vi "TCam_Config.vi"(8 "error in (no error)":errorcluster, 10 "crop?":bool, 11 "DataCluster in":T1={"Core"={"Current VI Reference"=refnum, "Close Panel on Exit?"=FALSE, "Exit"=FALSE, "Initialized?"=FALSE}, "Connections"={"cDAQ"={"Task"="", "Connected"=FALSE, "Active"=FALSE, "ID"=""}, "Camera"={"Session"="", "Connected"=FALSE, "Active"=FALSE, "Placeholder"=refnum}, "PSU"={"Port"="", "Connected"=FALSE, "Active"=FALSE}, "Arduino"={"Port"="", "Connected"=FALSE, "Active"=FALSE}}, "Data Acquisition"={"Setup"={"Label"="", "Operator"="", "Notes"="", "TempGrad"=1.0, "TargetTemp"=1.0, "Sample Volume"=1.0}, "Camera"={"Image"=refnum, "Save Image"=refnum, "Image Frequency"=20, "Rectangle"={"Left"=0, "Top"=0, "Right"=0, "Bottom"=0, "Rotation"=0.0}, "Calibration"={"Top Left"={"X"=0.0, "Y"=0.0}, "Top Right"={"X"=0.0, "Y"=0.0}, "Bottom Left"={"X"=0.0, "Y"=0.0}, "Bottom Right"={"X"=0.0, "Y"=0.0}, "Fixpoint"={"X"=0.0, "Y"=0.0}, "Scan Area"=0.0, "Fixpoint Area"=0.0, "Well Pixels"=[], "Valid"=FALSE}, "FocusPos"=0, "Display Mapping"=10, "Camera Mode"=10}, "Thermistor"={"Sample Size"=1, "Calibration"={"B0.100"=[], "R25"=[], "c"=[], "State"=[], "V_S"=5.0, "R_S"=100.0}, "Timing Mode"=14713}, "Partition"={"Data"=[], "Cell Label"="", "Cell Color"=0, "Height"=10, "Width"=16, "Grid"=[]}, "Queue"={"Size"=1, "Queue"=refnum}, "Sample Rate"=1, "Active"=FALSE, "Ready"=FALSE, "Graph Mode"=0, "Gradient Buffer"=2}, "Control"={"Sample Rate"=1, "PID gains"={"proportional gain (Kc)"=1.0, "integral time (Ti, min)"=0.01, "derivative time (Td, min)"=0.0}}, "Manual Temp Control"={"TargetTemp"=1.0, "Mode"=0, "Active"=FALSE}} {"Manual Temp Control"."Mode" items=["Cool", "Heat"]; "Manual Temp Control"."TargetTemp" min=-40.0 max=40.0 step=0.5 format="%#_g °C"; "Control"."PID gains"."derivative time (Td, min)" format="%.3f"; "Control"."PID gains"."integral time (Ti, min)" format="%.3f"; "Control"."PID gains"."proportional gain (Kc)" format="%.3f"; "Control"."Sample Rate" min=1 max=20 step=1 format="%.0f Samples/sec"; "Data Acquisition"."Gradient Buffer" min=2 max=30 step=1; "Data Acquisition"."Graph Mode" items=["Thermistor Temperature", "Camera Temperature"]; "Data Acquisition"."Thermistor"."Timing Mode" items=["Automatic"=16097, "High Resolution"=10195, "High Speed"=14712, "Best 50 Hz Rejection"=14713, "Best 60 Hz Rejection"=14714, "Custom"=10137]; "Data Acquisition"."Thermistor"."Calibration"."R_S" min=0.1 max=1000.0 format="%#_g kOhm"; "Data Acquisition"."Thermistor"."Calibration"."V_S" min=5.0 max=48.0 format="%#_g V"; "Data Acquisition"."Thermistor"."Calibration"."R25" min=0.1 max=1000.0 format="%#_g kOhm"; "Data Acquisition"."Thermistor"."Calibration"."B0.100" min=100.0 max=10000.0 format="%#_g K"; "Data Acquisition"."Thermistor"."Sample Size" min=1 max=200; "Data Acquisition"."Sample Rate" min=20 max=240 format="%.0f samples/min"; "Data Acquisition"."Queue"."Size" min=1 max=200; "Data Acquisition"."Camera"."Camera Mode" items=["Temperature Linear", "Signal Linear"]; "Data Acquisition"."Camera"."Display Mapping" items=["Default"=10, "Most Significant Bits"=11, "Full Dynamic"=12, "Downshift"=13, "Given Range"=14, "90% Dynamic"=15, "Given Percent Range"=16]; "Data Acquisition"."Camera"."Calibration"."Fixpoint"."Y" format="%.2f"; "Data Acquisition"."Camera"."Calibration"."Fixpoint"."X" format="%.2f"; "Data Acquisition"."Camera"."Calibration"."Top Left"."Y" format="%.2f"; "Data Acquisition"."Camera"."Calibration"."Top Left"."X" format="%.2f"; "Data Acquisition"."Camera"."Calibration"."Top Right"."Y" format="%.2f"; "Data Acquisition"."Camera"."Calibration"."Top Right"."X" format="%.2f"; "Data Acquisition"."Camera"."Calibration"."Bottom Left"."Y" format="%.2f"; "Data Acquisition"."Camera"."Calibration"."Bottom Left"."X" format="%.2f"; "Data Acquisition"."Camera"."Calibration"."Bottom Right"."Y" format="%.2f"; "Data Acquisition"."Camera"."Calibration"."Bottom Right"."X" format="%.2f"; "Data Acquisition"."Camera"."Rectangle"."Rotation" min=-90.0 max=90.0 step=1.0 format="%.2f"; "Data Acquisition"."Camera"."Rectangle"."Left" scale=0.0..1024.0; "Data Acquisition"."Camera"."Rectangle"."Right" scale=0.0..1024.0; "Data Acquisition"."Camera"."Image Frequency" min=1 max=60 step=1; "Data Acquisition"."Setup"."Sample Volume" min=0.0 max=500.0 format="%#_g µL"; "Data Acquisition"."Setup"."TargetTemp" min=-40.0 max=40.0 step=0.5 format="%#_g °C"; "Data Acquisition"."Setup"."TempGrad" min=-100.0 max=100.0 step=0.1 format="%#_g °C/min"}) -> (0 "error out":errorcluster, 3 "DataCluster out":T1={"Core"={"Current VI Reference"=refnum, "Close Panel on Exit?"=FALSE, "Exit"=FALSE, "Initialized?"=FALSE}, "Connections"={"cDAQ"={"Task"="", "Connected"=FALSE, "Active"=FALSE, "ID"=""}, "Camera"={"Session"="", "Connected"=FALSE, "Active"=FALSE, "Placeholder"=refnum}, "PSU"={"Port"="", "Connected"=FALSE, "Active"=FALSE}, "Arduino"={"Port"="", "Connected"=FALSE, "Active"=FALSE}}, "Data Acquisition"={"Setup"={"Label"="", "Operator"="", "Notes"="", "TempGrad"=1.0, "TargetTemp"=1.0, "Sample Volume"=1.0}, "Camera"={"Image"=refnum, "Save Image"=refnum, "Image Frequency"=20, "Rectangle"={"Left"=0, "Top"=0, "Right"=0, "Bottom"=0, "Rotation"=0.0}, "Calibration"={"Top Left"={"X"=0.0, "Y"=0.0}, "Top Right"={"X"=0.0, "Y"=0.0}, "Bottom Left"={"X"=0.0, "Y"=0.0}, "Bottom Right"={"X"=0.0, "Y"=0.0}, "Fixpoint"={"X"=0.0, "Y"=0.0}, "Scan Area"=0.0, "Fixpoint Area"=0.0, "Well Pixels"=[], "Valid"=FALSE}, "FocusPos"=0, "Display Mapping"=10, "Camera Mode"=10}, "Thermistor"={"Sample Size"=1, "Calibration"={"B0.100"=[], "R25"=[], "c"=[], "State"=[], "V_S"=5.0, "R_S"=100.0}, "Timing Mode"=14713}, "Partition"={"Data"=[], "Cell Label"="", "Cell Color"=0, "Height"=10, "Width"=16, "Grid"=[]}, "Queue"={"Size"=1, "Queue"=refnum}, "Sample Rate"=1, "Active"=FALSE, "Ready"=FALSE, "Graph Mode"=0, "Gradient Buffer"=2}, "Control"={"Sample Rate"=1, "PID gains"={"proportional gain (Kc)"=1.0, "integral time (Ti, min)"=0.01, "derivative time (Td, min)"=0.0}}, "Manual Temp Control"={"TargetTemp"=1.0, "Mode"=0, "Active"=FALSE}} {"Manual Temp Control"."Mode" items=["Cool", "Heat"]; "Manual Temp Control"."TargetTemp" min=-40.0 max=40.0 step=0.5 format="%#_g °C"; "Control"."PID gains"."derivative time (Td, min)" format="%.3f"; "Control"."PID gains"."integral time (Ti, min)" format="%.3f"; "Control"."PID gains"."proportional gain (Kc)" format="%.3f"; "Control"."Sample Rate" min=1 max=20 step=1 format="%.0f Samples/sec"; "Data Acquisition"."Gradient Buffer" min=2 max=30 step=1; "Data Acquisition"."Graph Mode" items=["Thermistor Temperature", "Camera Temperature"]; "Data Acquisition"."Thermistor"."Timing Mode" items=["Automatic"=16097, "High Resolution"=10195, "High Speed"=14712, "Best 50 Hz Rejection"=14713, "Best 60 Hz Rejection"=14714, "Custom"=10137]; "Data Acquisition"."Thermistor"."Calibration"."R_S" min=0.1 max=1000.0 format="%#_g kOhm"; "Data Acquisition"."Thermistor"."Calibration"."V_S" min=5.0 max=48.0 format="%#_g V"; "Data Acquisition"."Thermistor"."Calibration"."R25" min=0.1 max=1000.0 format="%#_g kOhm"; "Data Acquisition"."Thermistor"."Calibration"."B0.100" min=100.0 max=10000.0 format="%#_g K"; "Data Acquisition"."Thermistor"."Sample Size" min=1 max=200; "Data Acquisition"."Sample Rate" min=20 max=240 format="%.0f samples/min"; "Data Acquisition"."Queue"."Size" min=1 max=200; "Data Acquisition"."Camera"."Camera Mode" items=["Temperature Linear", "Signal Linear"]; "Data Acquisition"."Camera"."Display Mapping" items=["Default"=10, "Most Significant Bits"=11, "Full Dynamic"=12, "Downshift"=13, "Given Range"=14, "90% Dynamic"=15, "Given Percent Range"=16]; "Data Acquisition"."Camera"."Calibration"."Fixpoint"."Y" format="%.2f"; "Data Acquisition"."Camera"."Calibration"."Fixpoint"."X" format="%.2f"; "Data Acquisition"."Camera"."Calibration"."Top Left"."Y" format="%.2f"; "Data Acquisition"."Camera"."Calibration"."Top Left"."X" format="%.2f"; "Data Acquisition"."Camera"."Calibration"."Top Right"."Y" format="%.2f"; "Data Acquisition"."Camera"."Calibration"."Top Right"."X" format="%.2f"; "Data Acquisition"."Camera"."Calibration"."Bottom Left"."Y" format="%.2f"; "Data Acquisition"."Camera"."Calibration"."Bottom Left"."X" format="%.2f"; "Data Acquisition"."Camera"."Calibration"."Bottom Right"."Y" format="%.2f"; "Data Acquisition"."Camera"."Calibration"."Bottom Right"."X" format="%.2f"; "Data Acquisition"."Camera"."Rectangle"."Rotation" min=-90.0 max=90.0 step=1.0 format="%.2f"; "Data Acquisition"."Camera"."Rectangle"."Left" scale=0.0..1024.0; "Data Acquisition"."Camera"."Rectangle"."Right" scale=0.0..1024.0; "Data Acquisition"."Camera"."Image Frequency" min=1 max=60 step=1; "Data Acquisition"."Setup"."Sample Volume" min=0.0 max=500.0 format="%#_g µL"; "Data Acquisition"."Setup"."TargetTemp" min=-40.0 max=40.0 step=0.5 format="%#_g °C"; "Data Acquisition"."Setup"."TempGrad" min=-100.0 max=100.0 step=0.1 format="%#_g °C/min"})   [LabVIEW 2024]
uses:
  DataCluster.ctl
  <vilib>/userDefined/High Color/IMAQdx.ctl
  <vilib>/vision/Image Controls.llb/IMAQ Image.ctl
  <vilib>/vision/driver/IMAQdx.llb/IMAQdx Acquisition Mode.ctl
  05920238-52a0-44ea-981a-fd3a139130d6.vi
  <resource>/objmgr/imaqdx.rc
  <vilib>/vision/driver/NI_Vision_Acquisition_Software.lvlib
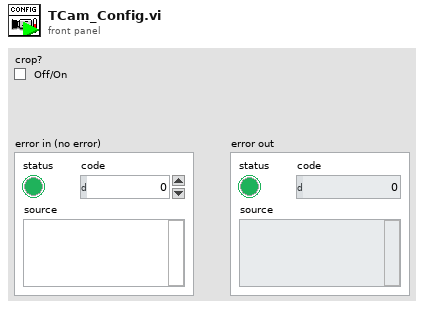
[diagram p1: front panel]
types:
  T1 = typedef "DataCluster.ctl" = cluster{"Core":cluster{"Current VI Reference":refnum<vi>, "Close Panel on Exit?":bool, "Exit":bool, "Initialized?":bool}, "Connections":cluster{"cDAQ":cluster{"Task":refnum<k21>, "Connected":bool, "Active":bool, "ID":string}, "Camera":cluster{"Session":T2, "Connected":bool, "Active":bool, "Placeholder":T3}, "PSU":cluster{"Port":refnum<visa-resource-name>, "Connected":bool, "Active":bool}, "Arduino":cluster{"Port":refnum<visa-resource-name>, "Connected":bool, "Active":bool}}, "Data Acquisition":cluster{"Setup":cluster{"Label":string, "Operator":string, "Notes":string, "TempGrad":dbl, "TargetTemp":dbl, "Sample Volume":dbl}, "Camera":cluster{"Image":T3, "Save Image":T3, "Image Frequency":i32, "Rectangle":T4, "Calibration":cluster{"Top Left":T5, "Top Right":T5, "Bottom Left":T5, "Bottom Right":T5, "Fixpoint":T5, "Scan Area":dbl, "Fixpoint Area":dbl, "Well Pixels":cluster{"X":i32, "Y":i32}[][], "Valid":bool}, "FocusPos":u32, "Display Mapping":u32, "Camera Mode":u32}, "Thermistor":cluster{"Sample Size":i32, "Calibration":cluster{"B0.100":dbl[], "R25":dbl[], "c":dbl[][], "State":bool[], "V_S":dbl, "R_S":dbl}, "Timing Mode":i32}, "Partition":cluster{"Data":string[][], "Cell Label":string, "Cell Color":u32, "Height":i32, "Width":i32, "Grid":string[][]}, "Queue":cluster{"Size":i32, "Queue":refnum<queue>}, "Sample Rate":i32, "Active":bool, "Ready":bool, "Graph Mode":u16, "Gradient Buffer":i32}, "Control":cluster{"Sample Rate":i32, "PID gains":cluster{"proportional gain (Kc)":dbl, "integral time (Ti, min)":dbl, "derivative time (Td, min)":dbl}}, "Manual Temp Control":cluster{"TargetTemp":dbl, "Mode":u16, "Active":bool}}
  T2 = typedef "IMAQdx.ctl" = refnum<k21>
  T3 = typedef "IMAQ Image.ctl" = refnum<image>
  T4 = typedef "IMAQ Rectangle" = cluster{"Left":i32, "Top":i32, "Right":i32, "Bottom":i32, "Rotation":dbl}
  T5 = typedef "IMAQ Point" = cluster{"X":sgl, "Y":sgl}
  T6 = typedef "NI_Vision_Acquisition_Software.lvlib/IMAQdx Acquisition Mode.ctl" = enum32{"One Shot", "Continuous"}
  T7 = typedef "Image Type" = u32
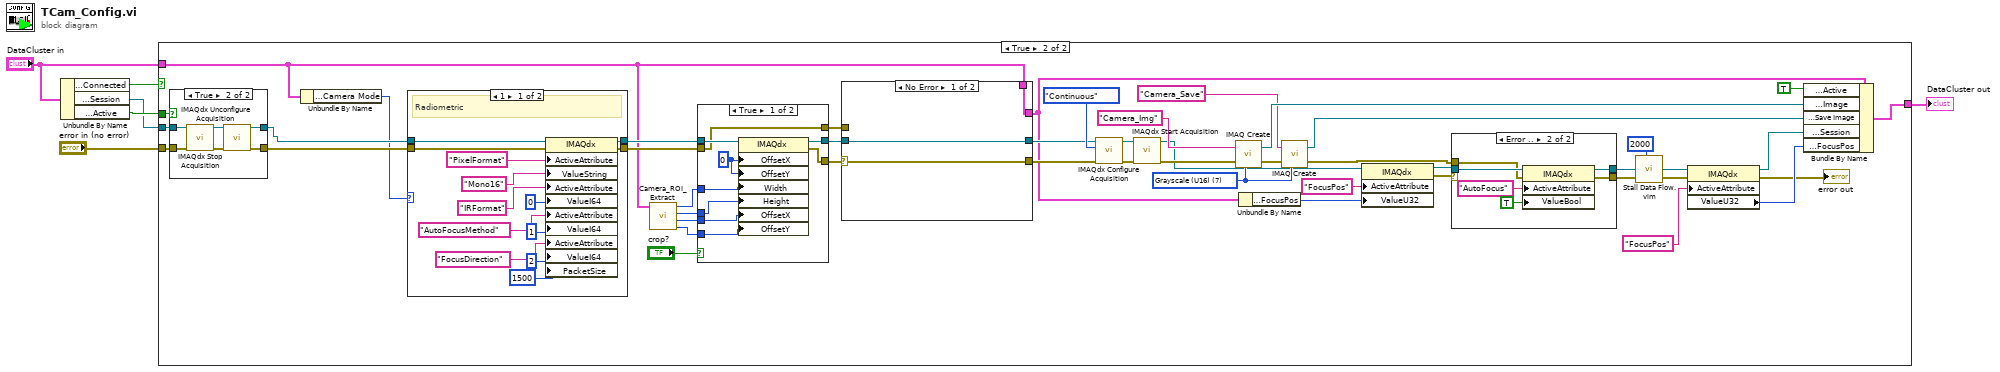
[diagram p0: block diagram]
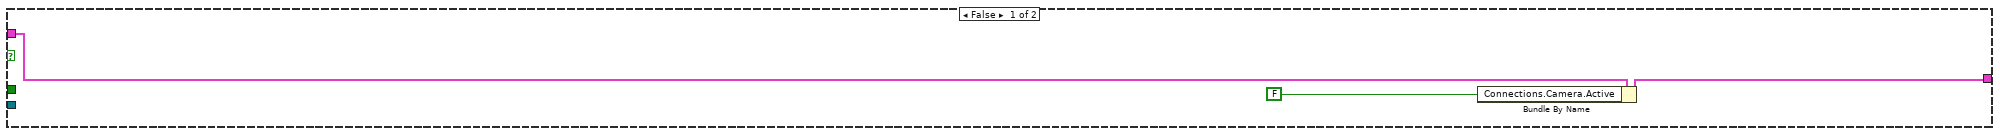
[diagram p2: hidden frame]
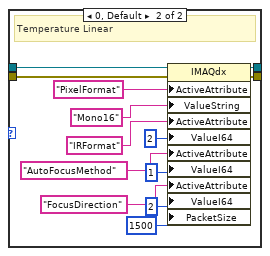
[diagram p3: hidden frame]
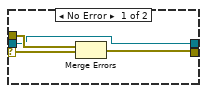
[diagram p4: hidden frame]
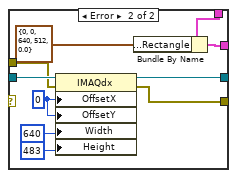
[diagram p6: hidden frame]
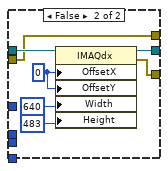
[diagram p7: hidden frame]
diagram:
  n1 = Unbundle By Name("DataCluster in") -> ("Connections.Camera.Connected"=w1:bool, "Connections.Camera.Session"=w2:T2, "Connections.Camera.Active"=w4:bool)
  n2 = case shown="True" w1 {
    tunnel: [w8 w55] -> w6
    tunnel: "DataCluster in" -> [w9 w11]
    tunnel: w4 -> [_ w44]
    tunnel: "error in (no error)" -> [_ w43]
    tunnel: w2 -> [_ w42]
    frame False {
      n3 = Bundle By Name(cluster=w9, "Connections.Camera.Active"=FALSE) -> (w8:T1)
    }
    frame True {
      w46 = T7 7 items=["Grayscale (U8)", "Grayscale (I16)", "Grayscale (SGL)", "Complex (CSG)", "RGB (U32)", "HSL (U32)", "RGB (U64)", "Grayscale (U16)"] ("Image Type")
      n4 = case shown="True" w44 {
        tunnel: w43 -> [w92 w97]
        tunnel: w42 -> [w93 w96]
        tunnel: [w93 w95] -> w32
        tunnel: [w92 w94] -> w29
        frame False {
        }
        frame True {
          n5 = call <vilib>:"IMAQdx Stop Acquisition.vi"("error in"=w97, "Session In"=w96) -> ("error out"=w98:errorcluster, "Session Out"=w99:T2)  [unwired: 8 in]
          n6 = call <vilib>:"IMAQdx Unconfigure Acquisition.vi"("error in"=w98, "Session In"=w99) -> ("error out"=w94:errorcluster, "Session Out"=w95:T2)  [unwired: 8 in]
        }
      }
      n7 = Unbundle By Name(w11) -> ("Data Acquisition.Camera.Camera Mode"=w10:u32)
      n8 = case shown="1" w10 {
        tunnel: w32 -> [w60 w73]
        tunnel: [w59 w72] -> w31
        tunnel: [w58 w71] -> w30
        tunnel: w29 -> [w57 w70]
        frame 1 {
          # "Radiometric"
          n9 = property class="IMAQdx"(reference=w60, error in=w57, "ActiveAttribute"="PixelFormat", "ValueString"="Mono16", "ActiveAttribute"="IRFormat", "ValueI64"=i64 0, "ActiveAttribute"="AutoFocusMethod", "ValueI64"=i64 1, "ActiveAttribute"="FocusDirection", "ValueI64"=i64 2, "PacketSize"=u32 1500) -> (reference out=w59:T2, error out=w58:errorcluster)
        }
        frame 0, Default {
          # "Temperature Linear"
          n10 = property class="IMAQdx"(reference=w73, error in=w70, "ActiveAttribute"="PixelFormat", "ValueString"="Mono16", "ActiveAttribute"="IRFormat", "ValueI64"=i64 2, "ActiveAttribute"="AutoFocusMethod", "ValueI64"=i64 1, "ActiveAttribute"="FocusDirection", "ValueI64"=i64 2, "PacketSize"=u32 1500) -> (reference out=w72:T2, error out=w71:errorcluster)
        }
      }
      n11 = call "Camera_ROI_Extract.vi"("input cluster"=w11) -> ("Offset Y"=w38:u32, "Offset X"=w39:u32, "Height"=w40:u32, "Width"=w41:u32)  [unwired: 7 in]
      n12 = case shown="True" "crop?" {
        tunnel: w31 -> [w121 w128]
        tunnel: w30 -> [w113 w122]
        tunnel: [w120 w127] -> w36
        tunnel: [w119 w126] -> w37
        tunnel: w41 -> [w117 _]
        tunnel: w40 -> [w116 _]
        tunnel: w39 -> [w115 _]
        tunnel: w38 -> [w114 _]
        tunnel: [w113 w122] -> w33
        frame True {
          w118 = u32 0 ("OffsetX")
          n13 = property class="IMAQdx"(reference=w121, "OffsetX"=w118, "OffsetY"=w118, "Width"=w117, "Height"=w116, "OffsetX"=w115, "OffsetY"=w114) -> (reference out=w120:T2, error out=w119:errorcluster)  [unwired: 1 in]
        }
        frame False {
          w125 = u32 0 ("OffsetX")
          n14 = property class="IMAQdx"(reference=w128, "OffsetX"=w125, "OffsetY"=w125, "Width"=u32 640, "Height"=u32 483) -> (reference out=w127:T2, error out=w126:errorcluster)  [unwired: 1 in]
        }
      }
      n15 = case shown="No Error" w37 {
        selector: w37 -> [w101 _]
        tunnel: w36 -> [w102 w109]
        tunnel: [w102 w108] -> w35
        tunnel: [w101 w107] -> w34
        tunnel: w11 -> [w100 w106]
        tunnel: [w100 w104] -> w28
        tunnel: w33 -> [_ w103]
        frame No Error {
        }
        frame Error {
          w110 = u32 0 ("OffsetX")
          n16 = property class="IMAQdx"(reference=w109, error in=w103, "OffsetX"=w110, "OffsetY"=w110, "Width"=u32 640, "Height"=u32 483) -> (reference out=w108:T2, error out=w107:errorcluster)
          n17 = Bundle By Name(cluster=w106, "Data Acquisition.Camera.Rectangle"=T4 {"Left"=0, "Top"=0, "Right"=640, "Bottom"=512, "Rotation"=0.0}) -> (w104:T1)
        }
      }
      n18 = call <vilib>:"IMAQdx Configure Acquisition.vi"("error in"=w34, "Continuous?"=IMAQdx_Acquisition_Mode."Continuous", "Session In"=w35) -> ("error out"=w12:errorcluster, "Session Out"=w13:T2)  [unwired: 7 in]
      n19 = call <vilib>:"IMAQdx Start Acquisition.vi"("error in"=w12, "Session In"=w13) -> ("error out"=w50:errorcluster, "Session Out"=w24:T2)  [unwired: 8 in]
      n20 = call "IMAQ Create"("Image Name"="Camera_Img", "Image Type"=w46, "error in (no error)"=w50) -> ("New Image"=w51:T3, "error out"=w48:errorcluster)  [unwired: 2 in]
      n21 = Unbundle By Name(w28) -> ("Data Acquisition.Camera.FocusPos"=w22:u32)
      n22 = call "IMAQ Create"("Image Name"="Camera_Save", "Image Type"=w46, "error in (no error)"=w48) -> ("New Image"=w47:T3, "error out"=w23:errorcluster)  [unwired: 2 in]
      n23 = property class="IMAQdx"(reference=w24, "ActiveAttribute"="FocusPos", "ValueU32"=w22) -> (reference out=w26:T2, error out=w25:errorcluster)  [unwired: 1 in]
      n24 = case shown="Error .." w25 {
        selector: w25 -> [w84 _]
        tunnel: [w82 w89] -> w15
        tunnel: w26 -> [w82 w88]
        tunnel: [w83 w87] -> w20
        tunnel: w23 -> [w85 w86]
        frame No Error {
          n25 = Merge Errors(w85, w84) -> (w83:errorcluster)
        }
        frame Error {
          n26 = property class="IMAQdx"(reference=w88, error in=w86, "ActiveAttribute"="AutoFocus", "ValueBool"=TRUE) -> (reference out=w89:T2, error out=w87:errorcluster)
        }
      }
      n27 = call "Stall Data Flow.vim"("value in"=w15, "milliseconds to wait"=u32 2000) -> ("value out"=w14:T2)  [unwired: 1 out]
      n28 = property class="IMAQdx"(reference=w14, error in=w20, "ActiveAttribute"="FocusPos") -> (reference out=w18:T2, error out=→"error out":errorcluster, "ValueU32"=w19:u32)
      n29 = Bundle By Name(cluster=w28, "Connections.Camera.Active"=TRUE, "Data Acquisition.Camera.Image"=w51, "Data Acquisition.Camera.Save Image"=w47, "Connections.Camera.Session"=w18, "Data Acquisition.Camera.FocusPos"=w19) -> (w55:T1)
    }
  }
  "DataCluster out" <- w6
